vi "prepare data table.vi"(8 "customViData":T1, 11 "New data":dbl[][](array[numeric])) -> (0 "customViData out":T1, 1 "plot data":cluster{"New data":dbl[], "New data":dbl[]}[](array[cluster]), 2 "chart data":dbl[][](array[numeric]), 3 "dataTable":string[][](table))   [LabVIEW 2018]
uses:
  customViData.ctl
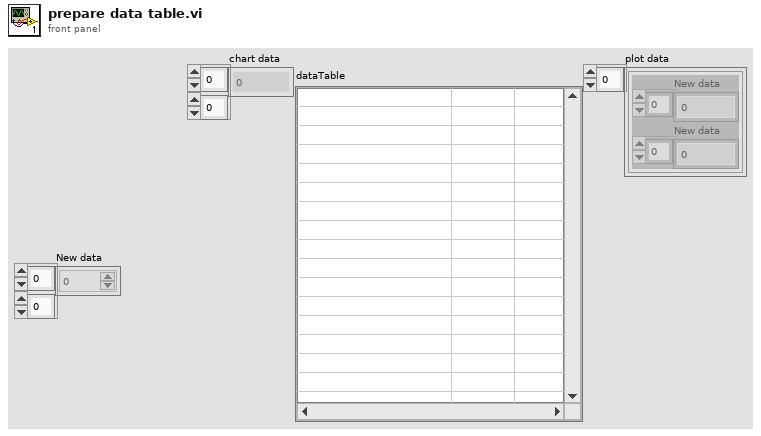
[diagram p1: front panel]
types:
  T1 = typedef "customViData.ctl" = cluster{"rigChannels":string[], "rigUnits":string[], "logging":bool, "plot":cluster{"X":u16[], "Y":u16[], "Y2":u16[]}, "updatePlot":bool, "chartRef":refnum<vi>, "livePlot":bool, "history":dbl[][], "channelCount":i32, "trendIndex":i32}
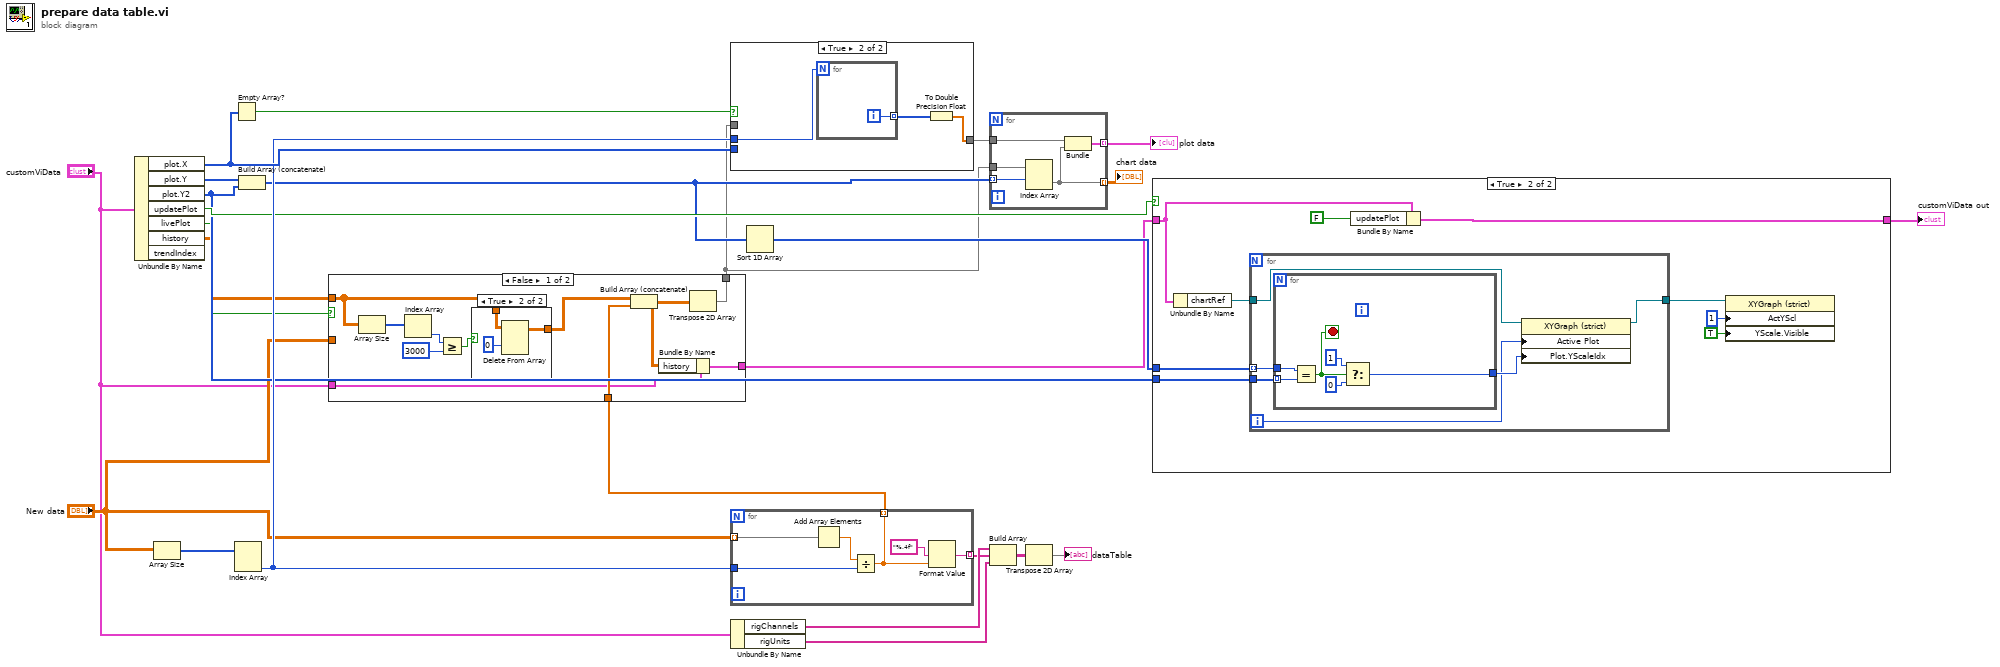
[diagram p0: block diagram]
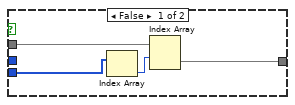
[diagram p5: hidden frame]
diagram:
  n1 = Unbundle By Name("customViData") -> ("plot.X"=w18:u16[], "plot.Y"=w19:u16[], "plot.Y2"=w9:u16[], "updatePlot"=w13:bool, "livePlot"=w7:bool, "history"=w6:dbl[][])  [unwired: 1 out]
  n2 = Array Size(array="New data") -> (size(s)=w25:i32[])
  n3 = Empty Array?(array=w18) -> (empty?=w17:bool)
  n4 = Index Array(array=w25) -> (element #2=w16:i32)  [unwired: 2 in, 1 out]
  n5 = Build Array (concatenate)(w19, w9) -> (w11:u16[])
  n6 = for {
    tunnel: "New data" -> [w31] mode=indexing
    tunnel: w16 -> [w29]
    tunnel: [w27] -> w23 mode=indexing
    tunnel: [w26] -> w4 mode=indexing
    n7 = Add Array Elements(numeric array=w31) -> (sum=w30:dbl)
    n8 = Divide(x=w30, y=w29) -> (x/y=w26:dbl)
    n9 = Format Value(format string="%.4f", value (0)=w26) -> (output string=w27:string)  [unwired: 1 in]
  }
  n10 = case shown="False" w7 {
    tunnel: w6 -> [w38 _]
    tunnel: "New data" -> [_ w47]
    tunnel: w4 -> [w42 _]
    tunnel: "customViData" -> [w34 w48]
    tunnel: [w33 w48] -> w2
    tunnel: [w32 w47] -> w1
    frame False {
      n11 = Array Size(array=w38) -> (size(s)=w41:i32[])
      n12 = Index Array(array=w41) -> (element=w40:i32)  [unwired: 1 in]
      n13 = Greater Or Equal?(x=w40, y=3000) -> (x >= y?=w36:bool)
      n14 = case shown="True" w36 {
        tunnel: w38 -> [w43 w46]
        tunnel: [w43 w45] -> w37
        frame False {
        }
        frame True {
          n15 = Delete From Array(array=w46, index (row)=0) -> (array with subset deleted=w45:dbl[][])  [unwired: 2 in, 1 out]
        }
      }
      n16 = Build Array (concatenate)(w37, w42) -> (w35:dbl[][])
      n17 = Bundle By Name(cluster=w34, "history"=w35) -> (w33:T1)
      n18 = Transpose 2D Array(2D array=w35) -> (transposed array=w32:dbl[][])
    }
    frame True {
    }
  }
  n19 = case shown="True" w17 {
    tunnel: [w51 w53] -> w20
    tunnel: w1 -> [w50 _]
    tunnel: w18 -> [w49 _]
    tunnel: w16 -> [_ w55]
    frame False {
      n20 = Index Array(array=w49) -> (element=w52:u16)  [unwired: 1 in]
      n21 = Index Array(array=w50, index (row)=w52) -> (element=w51:dbl[])  [unwired: 1 in]
    }
    frame True {
      n22 = for {
        N: w55 -> [_]
        tunnel: [w56] -> w54 mode=indexing
        i -> [w56]
      }
      n23 = To Double Precision Float(number=w54) -> (double precision float=w53:dbl[])
    }
  }
  n24 = Unbundle By Name("customViData") -> ("rigChannels"=w24:string[], "rigUnits"=w22:string[])
  n25 = Sort 1D Array(array=w11) -> (sorted array=w10:u16[])
  n26 = for {
    tunnel: w20 -> [w59]
    tunnel: w1 -> [w61]
    tunnel: w11 -> [w60] mode=indexing
    tunnel: [w58] -> w15 mode=indexing
    tunnel: [w57] -> w8 mode=indexing
    n27 = Index Array(array=w61, index (row)=w60) -> (element=w57:dbl[])  [unwired: 1 in]
    n28 = Bundle("New data"=w59, "New data"=w57) -> (w58:cluster{"New data":dbl[], "New data":dbl[]})  [unwired: 1 in]
  }
  "plot data" <- w15
  "chart data" <- w8
  n29 = Build Array(w24, w23, w22) -> (w21:string[][])
  n30 = Transpose 2D Array(2D array=w21) -> (transposed array=→"dataTable":string[][])
  n31 = case shown="True" w13 {
    tunnel: w2 -> [w62 w69]
    tunnel: [w62 w71] -> w12
    tunnel: w10 -> [_ w68]
    tunnel: w9 -> [_ w67]
    frame False {
    }
    frame True {
      n32 = Unbundle By Name(w69) -> ("chartRef"=w66:refnum<vi>)
      n33 = for {
        tunnel: w68 -> [w76] mode=indexing
        tunnel: w67 -> [w77]
        tunnel: w66 -> [w75]
        tunnel: [w73] -> w65
        i -> [w72]
        n34 = for {
          tunnel: w77 -> [w82] mode=indexing
          tunnel: w76 -> [w83]
          tunnel: [w78] -> w74
          stop <- w81 stop-if-true
          n35 = Equal?(x=w83, y=w82) -> (x = y?=w81:bool)
          n36 = Select(t=u32 1 ("Plot.Y Scale Index"), s=w81, f=u32 0 ("Plot.Y Scale Index")) -> (s? t:f=w78:u32)
        }
        n37 = property class="XYGraph (strict)"(reference=w75, "Active Plot"=w72, "Plot.YScaleIdx"=w74) -> (reference out=w73:refnum<vi>)  [unwired: 1 in, 1 out]
      }
      n38 = Bundle By Name(cluster=w69, "updatePlot"=FALSE) -> (w71:T1)
      n39 = property class="XYGraph (strict)"(reference=w65, "ActYScl"=1 ("Active Y Scale"), "YScale.Visible"=TRUE ("Y Scale.Visible")) -> ()  [unwired: 1 in, 2 out]
    }
  }
  "customViData out" <- w12
